vi "PipBoy_SendUEPipBoyCommand.vi"(8 "error in (no error)":errorcluster, 10 "Command":string="AcquirePipBoy", 11 "PipBoyData":T1) -> (0 "error out":errorcluster)   [LabVIEW 2014]
uses:
  ctls/PipBoy_PipBoyData.ctl
  ctls/PipBoy_ProcComm.ctl
  System.Windows.Forms
  ctls/PipBoy_PipBoyCommand.ctl
  ctls/PipBoy_Message.ctl
  modules/support/Message Queue/All Message Queues.ctl
  modules/support/Message Queue/Message Cluster.ctl
  ctls/PipBoy_FileConf.ctl
  ctls/PipBoy_PicComm.ctl
  ctls/PipBoy_GeneralParams.ctl
  ctls/PipBoy_Pages.ctl
  modules/support/Message Queue/Message Queue.lvlib
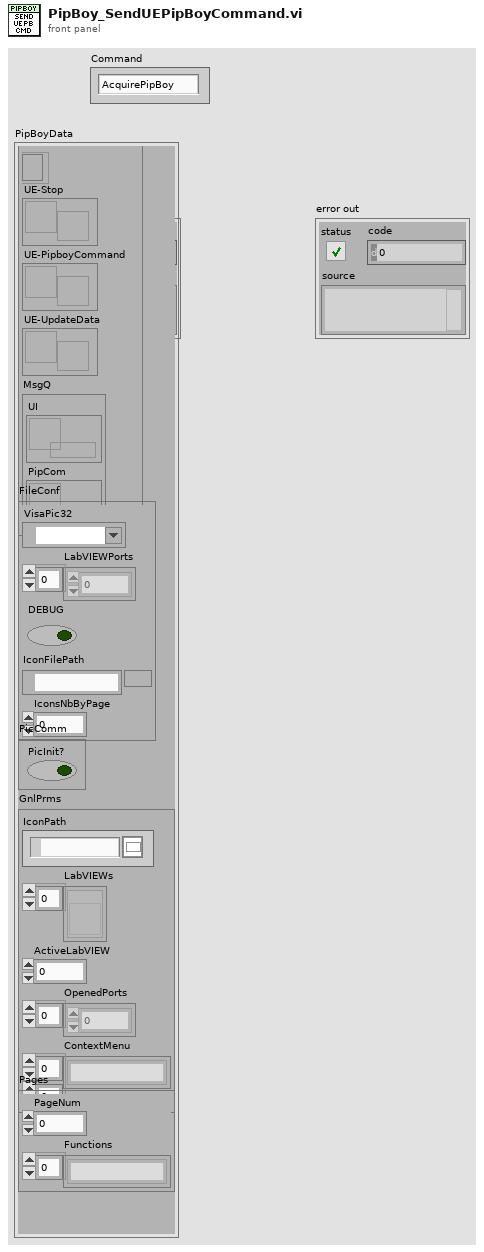
[diagram p1: front panel]
types:
  T1 = typedef "PipBoy_PipBoyData.ctl" = cluster{"ProcComm":T2, "FileConf":T4, "PicComm":T5, "GnlPrms":T6, "Pages":T7}
  T2 = typedef "PipBoy_ProcComm.ctl" = cluster{"NotifyIconRef":refnum<k24>, "UE-Stop":refnum<user-event>, "UE-PipboyCommand":refnum<user-event>, "UE-UpdateData":refnum<user-event>, "MsgQ":T3}
  T3 = typedef "Message Queue.lvlib/All Message Queues.ctl" = cluster{"UI":refnum<queue>, "PipCom":refnum<queue>}
  T4 = typedef "PipBoy_FileConf.ctl" = cluster{"VisaPic32":refnum<visa-resource-name>, "LabVIEWPorts":u16[], "DEBUG":bool, "IconFilePath":path, "IconsNbByPage":i32}
  T5 = typedef "PipBoy_PicComm.ctl" = cluster{"PicInit?":bool}
  T6 = typedef "PipBoy_GeneralParams.ctl" = cluster{"IconPath":path, "LabVIEWs":refnum<vi>[], "ActiveLabVIEW":i32, "OpenedPorts":u16[], "ContextMenu":string[][]}
  T7 = typedef "PipBoy_Pages.ctl" = cluster{"PageNum":i32, "Functions":string[]}
  T8 = typedef "PipBoy_PipBoyCommand.ctl" = cluster{"Name":string}
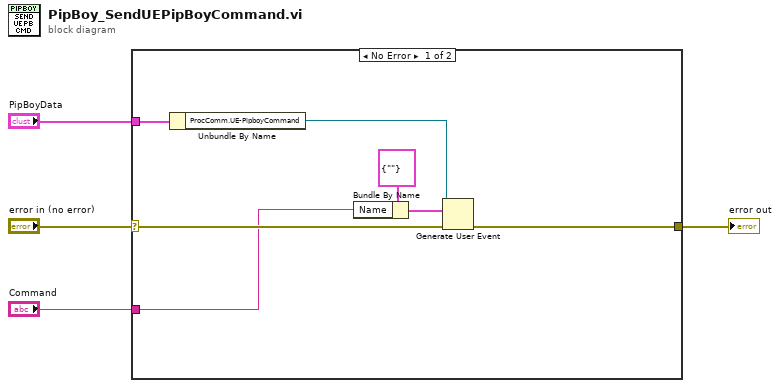
[diagram p0: block diagram]
diagram:
  n1 = case shown="No Error" "error in (no error)" {
    selector: "error in (no error)" -> [w11 w12]
    tunnel: "PipBoyData" -> [w9 _]
    tunnel: "Command" -> [w6 _]
    tunnel: [w10 w12] -> w2
    frame No Error {
      n2 = Unbundle By Name(w9) -> ("ProcComm.UE-PipboyCommand"=w7:refnum<user-event>)
      n3 = Bundle By Name(cluster=T8 {"Name"=""} ("event data"), "Name"=w6) -> (w5:T8)
      n4 = Generate User Event(user event=w7, event data cluster=w5, error in=w11) -> (error out=w10:errorcluster)  [unwired: 1 in, 1 out]
    }
    frame Error {
    }
  }
  "error out" <- w2
